vi "Proxy_Remove VI Packages from VIPM Package Library_vipm_api.vi"(8 "error in (no error)":errorcluster, 9 "LabVIEW Version":string, 10 "Package Names to Remove":string[](array[string])) -> (0 "error out":errorcluster, 2 "Packages Removed":string[](array[string]))   [LabVIEW 2017, in "CL_G3_VIPMUtilities.lvlib"]
doc: "This VI dynamically invokes the VIPM API with a timeout. VPIM will randomly hang for reasons we don't understand. This vi detects if there is a hang, force closes VIPM and then restarts it."
uses:
  CL_G3_VIPMUtilities.lvlib
  Proxy States.ctl
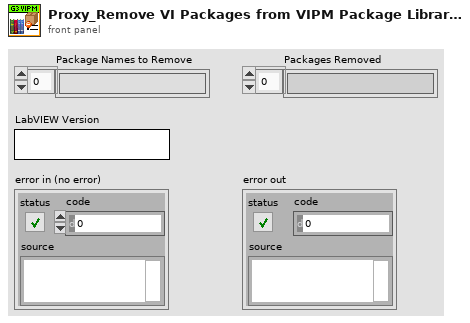
[diagram p1: front panel]
types:
  T1 = typedef "CL_G3_VIPMUtilities.lvlib/Proxy States.ctl" = enum16{"Initialize", "Start Proxy", "Wait on Proxy", "Force Quit VIPM", "Close Proxy"}
  T2 = cluster{"Proxy Path":path, "LabVIEW Version":string, "error out":errorcluster, "Proxy VI Ref":refnum<vi>, "Restart Count":i32, "Maximum restart tries":i32, "Package Names to Remove":string[], "Packages Removed":string[]}
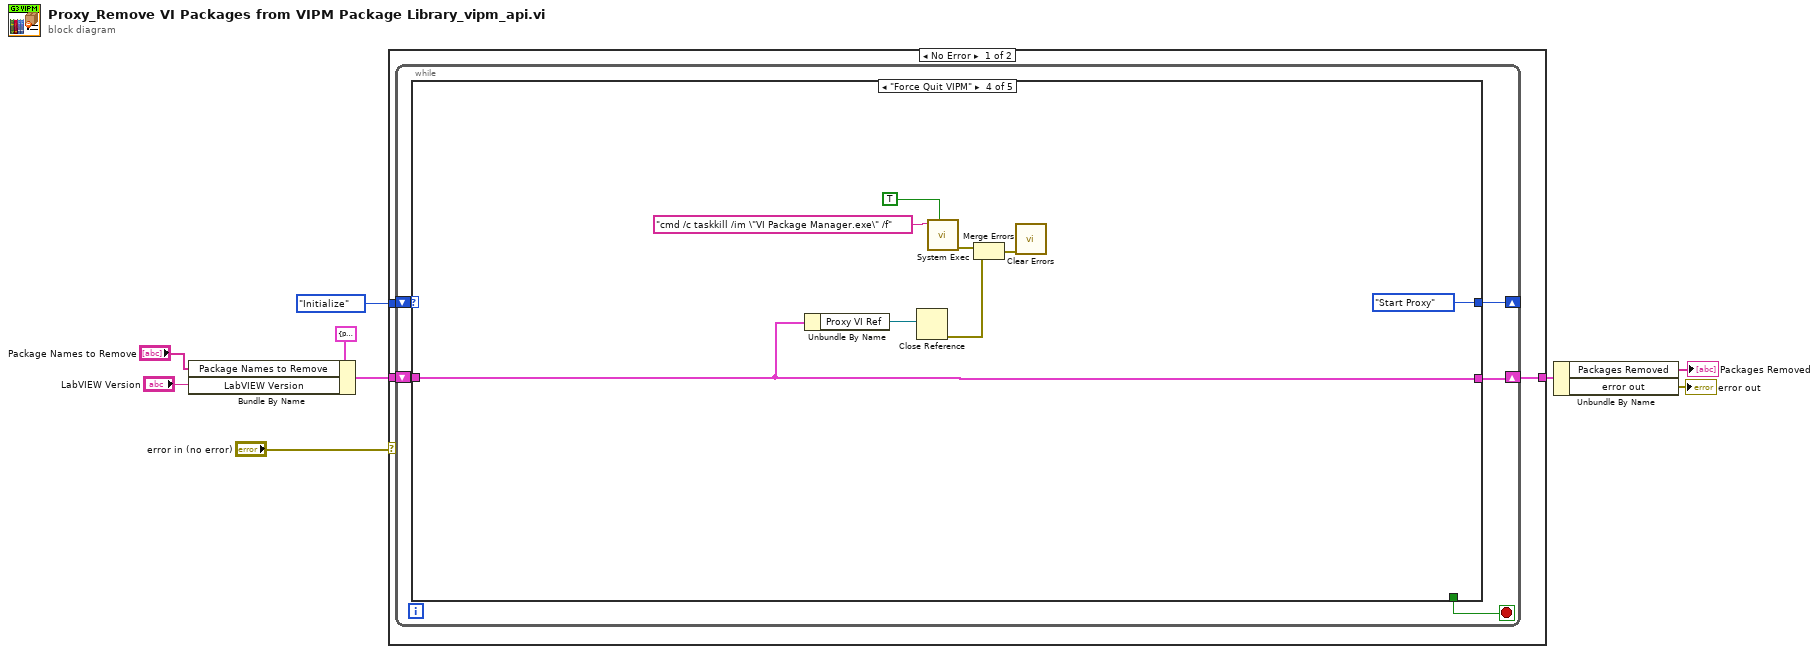
[diagram p0: block diagram]
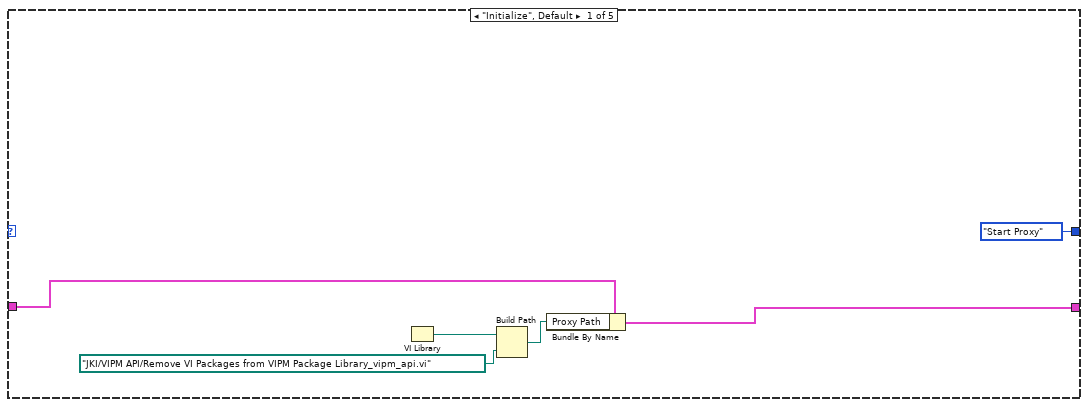
[diagram p2: hidden frame]
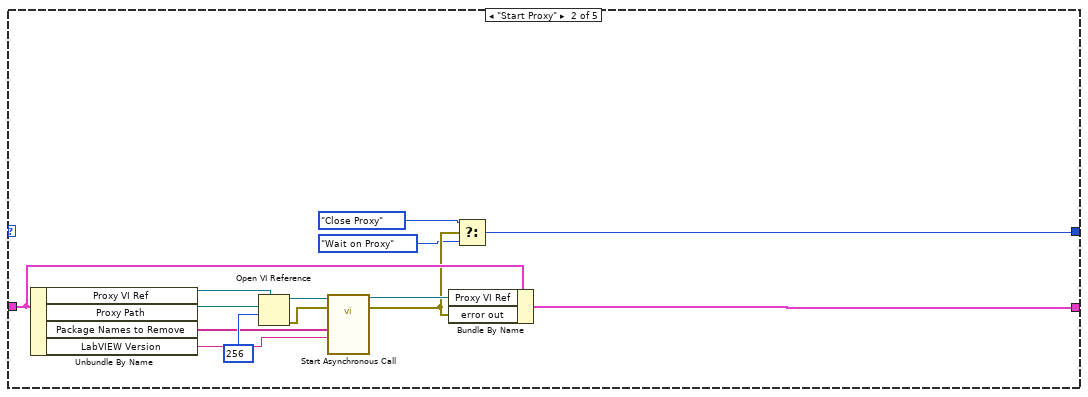
[diagram p3: hidden frame]
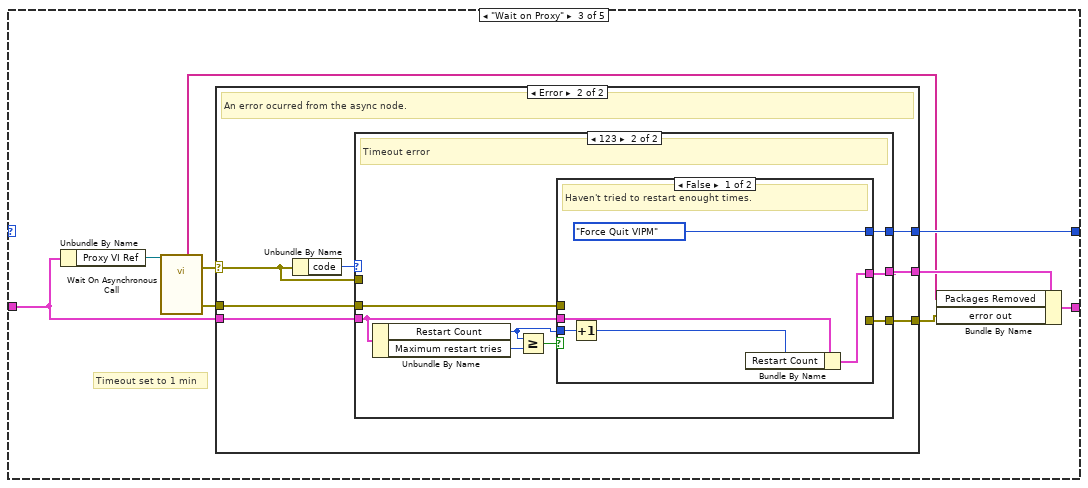
[diagram p4: hidden frame]
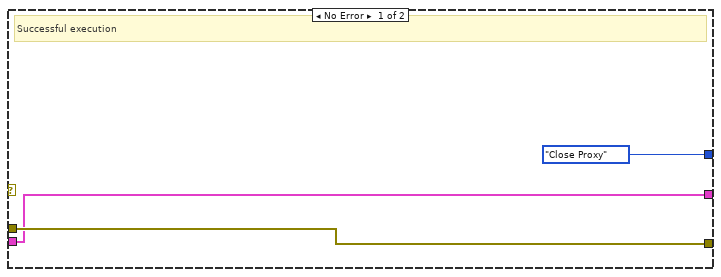
[diagram p5: hidden frame]
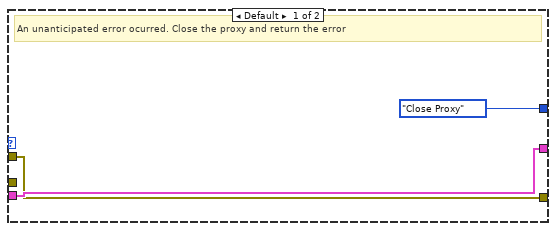
[diagram p6: hidden frame]
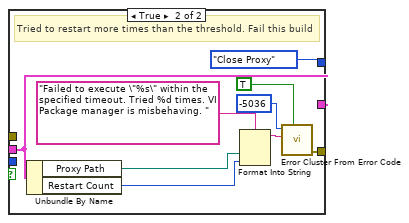
[diagram p7: hidden frame]
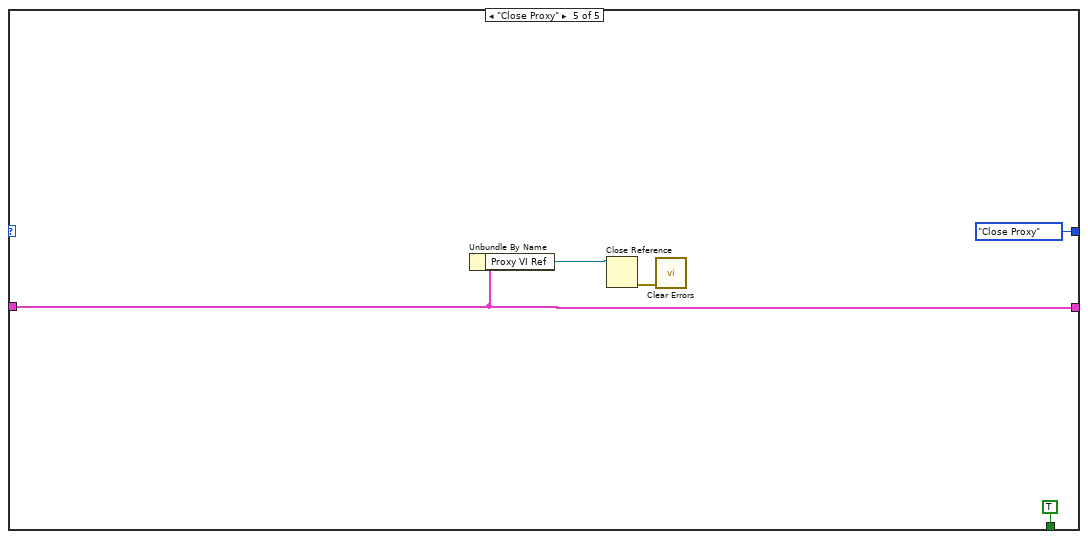
[diagram p8: hidden frame]
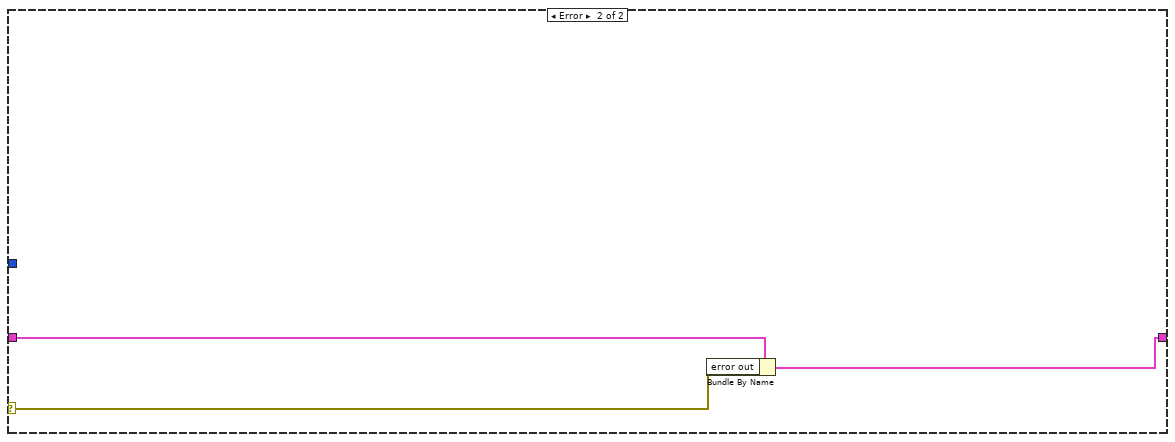
[diagram p9: hidden frame]
diagram:
  n1 = Bundle By Name(cluster=T2 {"Proxy Path"=path "", "LabVIEW Version"="", "error out"={"status"=FALSE, "code"=0, "source"=""}, "Proxy VI Ref"=refnum, "Restart Count"=0, "Maximum restart tries"=5, "Package Names to Remove"=[], "Packages Removed"=[]}, "Package Names to Remove"="Package Names to Remove", "LabVIEW Version"="LabVIEW Version") -> (w8:T2)
  n2 = case shown="No Error" "error in (no error)" {
    selector: "error in (no error)" -> [_ w96]
    tunnel: w8 -> [w12 w97]
    tunnel: Proxy_States."Initialize" -> [w11 _]
    tunnel: [w10 w95] -> w4
    frame No Error {
      n3 = while {
        shift-right: [w15] -> _
        shift-left: w11 -> [w17]
        shift-right: [w14] -> w10
        shift-left: w12 -> [w16]
        stop <- w13 stop-if-true
        n4 = case shown="\"Force Quit VIPM\"" w17 {
          tunnel: [w22 w32 w46 w83 w92] -> w14
          tunnel: w16 -> [w23 w37 w42 w83 w92]
          tunnel: [Proxy_States."Start Proxy" w27 w40 Proxy_States."Start Proxy" Proxy_States."Close Proxy"] -> w15
          tunnel: [_ _ _ _ TRUE] -> w13
          frame "Initialize", Default {
            n5 = VI Library() -> (path=w20:path)
            n6 = Build Path(base path=w20, name or relative path=path "JKI/VIPM API/Remove VI Packages from VIPM Package Library_vipm_api.vi" ("Proxy Path")) -> (appended path=w18:path)
            n7 = Bundle By Name(cluster=w23, "Proxy Path"=w18) -> (w22:T2)
          }
          frame "Start Proxy" {
            n8 = Unbundle By Name(w37) -> ("Proxy VI Ref"=w26:refnum<vi>, "Proxy Path"=w36:path, "Package Names to Remove"=w24:string[], "LabVIEW Version"=w34:string)
            n9 = Open VI Reference(type specifier VI Refnum (for type only)=w26, vi path=w36, options=256) -> (vi reference=w35:refnum<vi>, error out=w33:errorcluster)  [unwired: 3 in]
            n10 = call-by-ref "Start Asynchronous Call"(reference=w35, error in=w33, "LabVIEW Version"=w34, "Package Names to Remove"=w24) -> (reference out=w31:refnum<vi>, error out=w30:errorcluster)  [unwired: 8 in, 2 out]
            n11 = Bundle By Name(cluster=w37, "Proxy VI Ref"=w31, "error out"=w30) -> (w32:T2)
            n12 = Select(t=Proxy_States."Close Proxy", s=w30, f=Proxy_States."Wait on Proxy") -> (s? t:f=w27:T1)
          }
          frame "Wait on Proxy" {
            # "Timeout set to 1 min"
            n13 = Unbundle By Name(w42) -> ("Proxy VI Ref"=w38:refnum<vi>)
            n14 = call-by-ref "Wait On Asynchronous Call"(reference=w38) -> (error out=w43:errorcluster, 0:"error out"=w44:errorcluster, "Packages Removed"=w39:string[])  [unwired: 11 in, 1 out]
            n15 = case shown="Error" w43 {
              selector: w43 -> [_ w50]
              tunnel: [w49 w53] -> w45
              tunnel: w44 -> [w49 w52]
              tunnel: w42 -> [w47 w55]
              tunnel: [w47 w54] -> w41
              tunnel: [Proxy_States."Close Proxy" w51] -> w40
              frame No Error {
                # "Successful execution"
              }
              frame Error {
                # "An error ocurred from the async node."
                n16 = Unbundle By Name(w50) -> ("code"=w56:i32)
                n17 = case shown="123" w56 {
                  tunnel: w55 -> [w59 w67]
                  tunnel: [w59 w66] -> w54
                  tunnel: [w57 w62] -> w53
                  tunnel: w52 -> [_ w61]
                  tunnel: [Proxy_States."Close Proxy" w63] -> w51
                  tunnel: w50 -> [w57 _]
                  frame Default {
                    # "An unanticipated error ocurred. Close the proxy and return the error"
                  }
                  frame 123 {
                    # "Timeout error"
                    n18 = Unbundle By Name(w67) -> ("Restart Count"=w65:i32, "Maximum restart tries"=w60:i32)
                    n19 = Greater Or Equal?(x=w65, y=w60) -> (x >= y?=w64:bool)
                    n20 = case shown="False" w64 {
                      tunnel: w67 -> [w72 w75]
                      tunnel: [w71 w75] -> w66
                      tunnel: w65 -> [w68 _]
                      tunnel: [Proxy_States."Force Quit VIPM" Proxy_States."Close Proxy"] -> w63
                      tunnel: [_ w79] -> w62
                      tunnel: w61 -> [_ _]
                      frame False {
                        # "Haven't tried to restart enought times."
                        n21 = Increment(x=w68) -> (x+1=w69:i32)
                        n22 = Bundle By Name(cluster=w72, "Restart Count"=w69) -> (w71:T2)
                      }
                      frame True {
                        # "Tried to restart more times than the threshold. Fail this build"
                        n23 = Unbundle By Name(w75) -> ("Proxy Path"=w74:path, "Restart Count"=w73:i32)
                        n24 = Format Into String(format string="Failed to execute \"%s\" within the specified timeout. Tried %d times. VI Package manager is misbehaving. ", w74, w73) -> (resulting string=w76:string)  [unwired: 2 in, 1 out]
                        n25 = call <vilib>:"Error Cluster From Error Code.vi"("show call chain? (False)"=TRUE, "error message (\"\")"=w76, "error code (0)"=-5036) -> ("error out"=w79:errorcluster)  [unwired: 6 in]
                      }
                    }
                  }
                }
              }
            }
            n26 = Bundle By Name(cluster=w41, "Packages Removed"=w39, "error out"=w45) -> (w46:T2)
          }
          frame "Force Quit VIPM" {
            n27 = Unbundle By Name(w83) -> ("Proxy VI Ref"=w86:refnum<vi>)
            n28 = Close Reference(reference=w86) -> (error out=w84:errorcluster)  [unwired: 1 in]
            n29 = call <vilib>:"System Exec.vi"("run minimized? (F)"=TRUE, "command line"="cmd /c taskkill /im \"VI Package Manager.exe\" /f") -> ("error out"=w87:errorcluster)  [unwired: 6 in, 3 out]
            n30 = Merge Errors(w87, w84) -> (w85:errorcluster)
            n31 = call <vilib>:"Clear Errors.vi"("error in (no error)"=w85) -> ()  [unwired: 5 in, 2 out]
          }
          frame "Close Proxy" {
            n32 = Unbundle By Name(w92) -> ("Proxy VI Ref"=w91:refnum<vi>)
            n33 = Close Reference(reference=w91) -> (error out=w90:errorcluster)  [unwired: 1 in]
            n34 = call <vilib>:"Clear Errors.vi"("error in (no error)"=w90) -> ()  [unwired: 5 in, 2 out]
          }
        }
      }
    }
    frame Error {
      n35 = Bundle By Name(cluster=w97, "error out"=w96) -> (w95:T2)
    }
  }
  n36 = Unbundle By Name(w4) -> ("Packages Removed"=→"Packages Removed":string[], "error out"=→"error out":errorcluster)
